vi "HO3_1.vi"() -> ()   [LabVIEW 2020]
panel:
  out "Message":string
  out "Contact Indicator":T1={"First Name"="", "Last Name"="", "Birthday"=timestamp(61200.46228170395 s since 1904-01-01), "Favorite"=FALSE, "\nAge"=""} {"Birthday" format="%<%x>T"}
  out "Birthday":string
  out "Current Time":string
  in  "Contact":T1={"First Name"="", "Last Name"="", "Birthday"=timestamp(61200.46228170395 s since 1904-01-01), "Favorite"=FALSE, "\nAge"=""} {"Birthday" format="%<%x>T"}
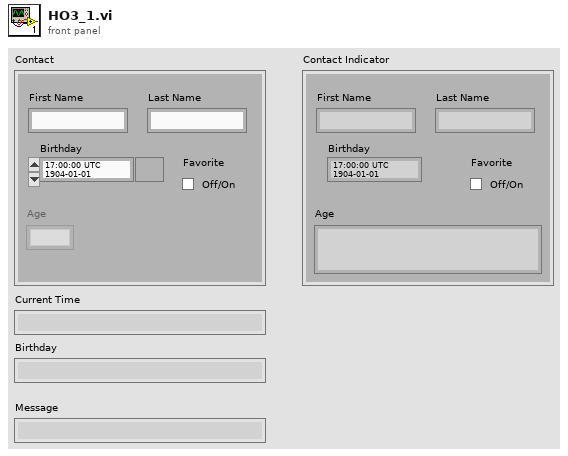
[diagram p1: front panel]
types:
  T1 = cluster{"First Name":string, "Last Name":string, "Birthday":timestamp, "Favorite":bool, "\nAge":string}
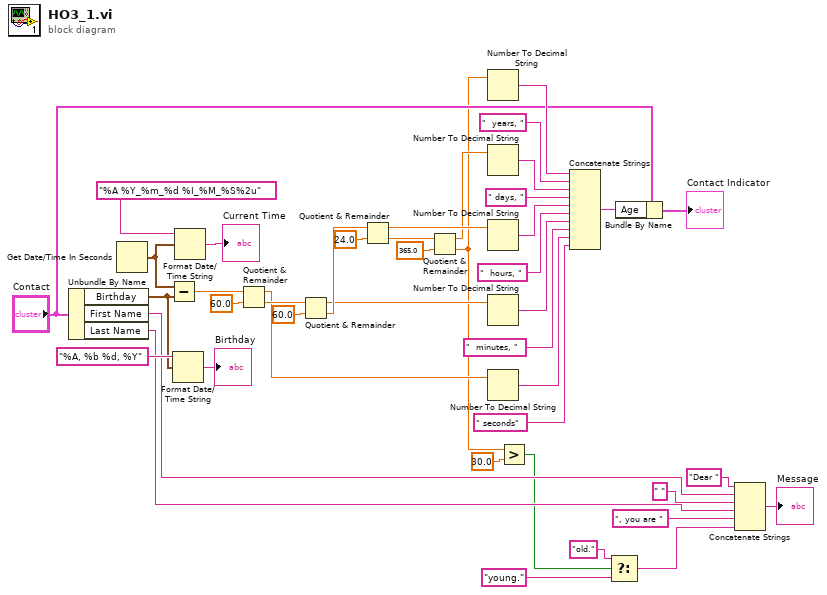
[diagram p0: block diagram]
diagram:
  n1 = Unbundle By Name("Contact") -> ("Birthday"=w17:timestamp, "First Name"=w10:string, "Last Name"=w8:string)
  n2 = Get Date/Time In Seconds() -> (seconds since 1Jan1904=w16:timestamp)
  n3 = Subtract(x=w16, y=w17) -> (x-y=w39:dbl)
  n4 = Format Date/Time String(time format string (%c)="%A, %b %d, %Y", seconds (now)=w17) -> (date/time string=→"Birthday":string)  [unwired: 1 in]
  n5 = Format Date/Time String(time format string (%c)="%A %Y_%m_%d %I_%M_%S%2u", seconds (now)=w16) -> (date/time string=→"Current Time":string)  [unwired: 1 in]
  n6 = Quotient & Remainder(x=w39, y=60.0) -> (x-y*floor(x/y)=w31:dbl, floor(x/y)=w37:dbl)
  n7 = Quotient & Remainder(x=w37, y=60.0) -> (x-y*floor(x/y)=w30:dbl, floor(x/y)=w35:dbl)
  n8 = Quotient & Remainder(x=w35, y=24.0) -> (x-y*floor(x/y)=w29:dbl, floor(x/y)=w33:dbl)
  n9 = Quotient & Remainder(x=w33, y=365.0) -> (x-y*floor(x/y)=w28:dbl, floor(x/y)=w5:dbl)
  n10 = Number To Decimal String(number=w5) -> (decimal integer string=w27:string)  [unwired: 1 in]
  n11 = Number To Decimal String(number=w28) -> (decimal integer string=w25:string)  [unwired: 1 in]
  n12 = Number To Decimal String(number=w29) -> (decimal integer string=w23:string)  [unwired: 1 in]
  n13 = Number To Decimal String(number=w30) -> (decimal integer string=w21:string)  [unwired: 1 in]
  n14 = Number To Decimal String(number=w31) -> (decimal integer string=w19:string)  [unwired: 1 in]
  n15 = Greater?(x=w5, y=30.0) -> (0:w3:bool)
  n16 = Concatenate Strings(w27, "  years, ", w25, " days, ", w23, "  hours, ", w21, "  minutes, ", w19, " seconds") -> (w14:string)
  n17 = Select(t="old.", s=w3, f="young.") -> (s? t:f=w6:string)
  n18 = Bundle By Name(cluster="Contact", "Age"=w14) -> (→"Contact Indicator":T1)
  n19 = Concatenate Strings("Dear ", w10, " ", w8, ", you are ", w6) -> (→"Message":string)
